vi "Write Parent Ref.vi"(8 "error in (no error)":errorcluster, 10 "Parent in":refnum<vi>, 11 "Transform Ref in":refnum<vi>) -> (0 "error out":errorcluster, 3 "Transform Ref out":refnum<vi>)   [LabVIEW 2022 SP3, in "Transform.lvclass"]
uses:
  Transform.lvclass
  Transform.lvclass/Transform.ctl
  D:/Programowanie/Studia/Labview/CollisionSimulator/Project/Engine/Objects/Components/Component/Component.lvclass
  D:/Programowanie/Studia/Labview/CollisionSimulator/Project/Engine/Objects/Components/Transform/Transform.lvclass
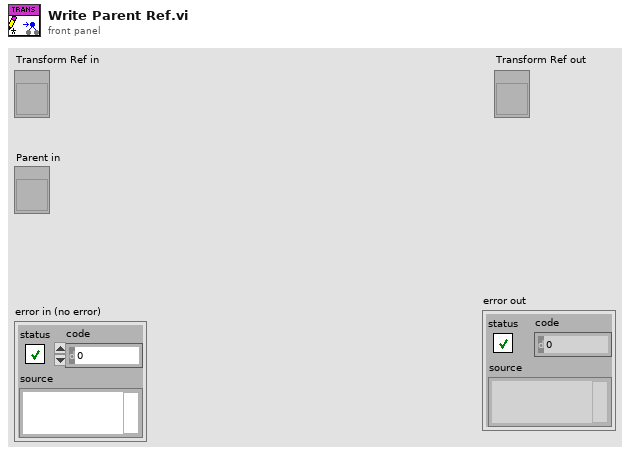
[diagram p1: front panel]
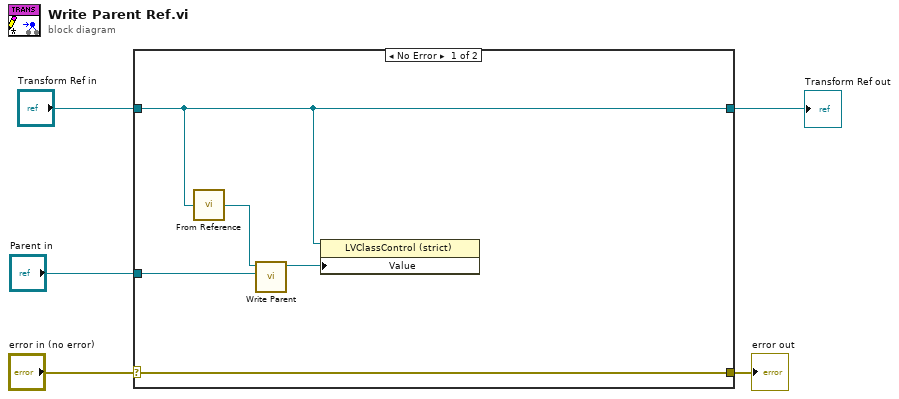
[diagram p0: block diagram]
diagram:
  n1 = case shown="No Error" "error in (no error)" {
    selector: "error in (no error)" -> [w10 w12]
    tunnel: [w10 w12] -> w4
    tunnel: [w7 w11] -> w2
    tunnel: "Transform Ref in" -> [w7 w11]
    tunnel: "Parent in" -> [w9 _]
    frame No Error {
      n2 = call "From Reference.vi"("Transform Ref in"=w7) -> ("Transform out"=w8:refnum<class "Transform.lvclass">)
      n3 = call "Write Parent.vi"("Parent"=w9, "Transform in"=w8) -> ("Transform out"=w6:refnum<class "Transform.lvclass">)  [unwired: 8 in, 1 out]
      n4 = property class="LVClassControl (strict)"(reference=w7, "Value"=w6) -> ()  [unwired: 1 in, 2 out]
    }
    frame Error {
    }
  }
  "error out" <- w4
  "Transform Ref out" <- w2
